vi "WriteData.vi"(8 "error in":errorcluster, 11 "refnum in":refnum<file>) -> (0 "error out":errorcluster, 3 "refnum out":refnum<file>)   [LabVIEW 2017]
doc: "Logs data to csv file on roborio"
uses:
  Robot Global Data.vi
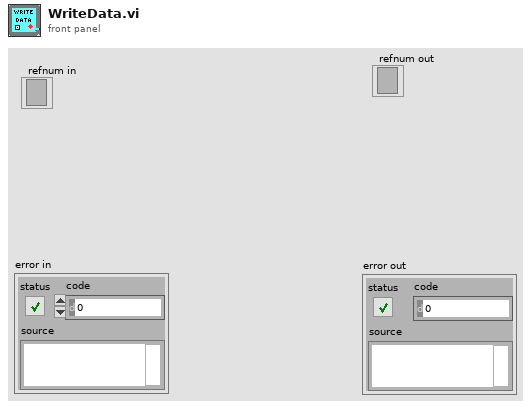
[diagram p1: front panel]
types:
  T1 = typedef "WPI_DriverStationRobotMode2.ctl" = enum16{"Autonomous Disabled", "Autonomous Enabled", "Teleop Disabled", "Teleop Enabled", "Disconnected", "Finish", "Test Disabled", "Test Enabled", "Emergency Stopped"}
  T2 = typedef "Z900_navX_Flags_OpStatusTypeDef.ctl" = u8
  T3 = typedef "Z900_navX_Flags_CalibrationStatusTypeDef.ctl" = u8
  T4 = cluster{"Update Rate Hz":u8, "Accelerometer Full-Scale Range":u8, "Gyro Full-Scale Range":u16, "OP Status":T2, "Calibration Status":T3, "Sensor Status":cluster{"MOVING":bool, "YAW_STABLE":bool, "MAG_DISTURBANCE":bool, "ALTITUDE_VALID":bool, "SEALEVEL_PRESS_SET":bool, "FUSED_HEADING_VALID":bool}, "Self Test Status":cluster{"Gyro Passed":bool, "Accel Passed":bool, "Mag Passed":bool, "Baro Passed":bool, "Complete":bool}}
  T5 = cluster{"Yaw":dbl, "Roll":dbl, "Pitch":dbl, "Heading":dbl, "Fused Heading":dbl}
  T6 = cluster{"LinearAcceleration X":dbl, "LinearAcceleration Y":dbl, "LinearAcceleration Z":dbl}
  T7 = cluster{"MOVING":bool, "YAW_STABLE":bool, "MAG_DISTURBANCE":bool, "ALTITUDE_VALID":bool, "SEALEVEL_PRESS_SET":bool, "FUSED_HEADING_VALID":bool}
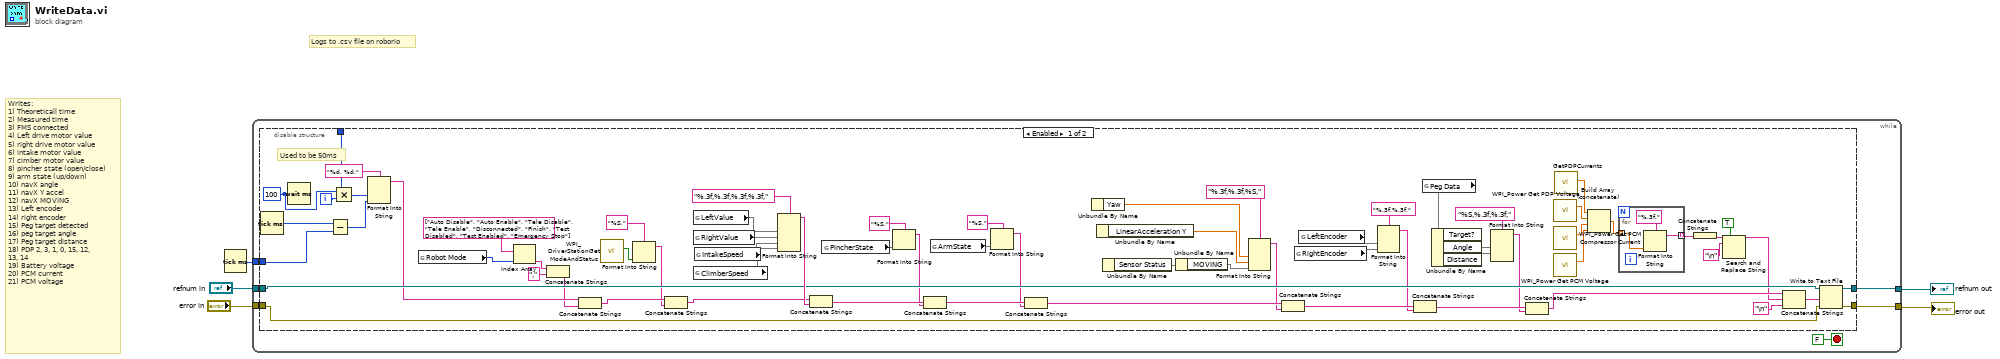
[diagram p0: block diagram]
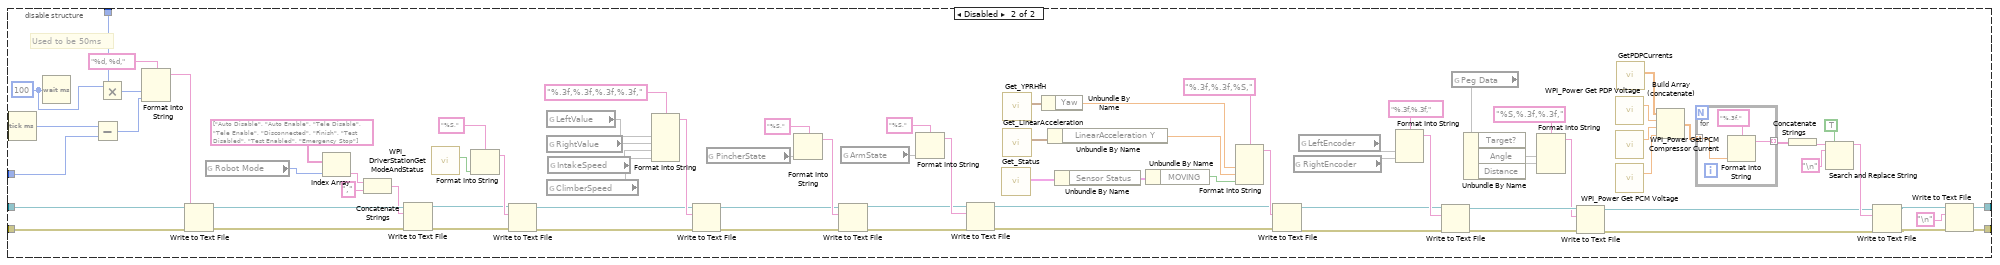
[diagram p2: hidden frame]
diagram:
  # "Logs to .csv file on roborio"
  # "Writes:\n1) Theoreticall time\n2) Measured time\n3) FMS connected\n4) Left drive motor value\n5) right drive motor value\n6) intake motor value\n7) cimber motor value\n8) pincher state (open/close)\n9) arm state (up/down)\n10) navX angle\n11) navX Y accel\n12) navX MOVING\n13) Left encoder\n14) right encoder\n15) Peg target detected\n16) peg target angle\n17) Peg target distance\n18) PDP 2, 3, 1, 0, 15, 12,\n13, 14\n19) Battery voltage\n20) PCM current\n21) PCM voltage"
  n1 = Tick Count (ms)() -> (millisecond timer value=w1:u32)
  n2 = while {
    tunnel: "error in" -> [w10]
    tunnel: "refnum in" -> [w9]
    tunnel: [w7] -> w3
    tunnel: [w8] -> w2
    tunnel: w1 -> [w6]
    i -> [w11]
    stop <- FALSE stop-if-true
    n3 = disable-structure shown="Enabled" {
      disable-tunnel: w11 -> [w80 w165]
      disable-tunnel: w10 -> [w30 w162]
      disable-tunnel: w9 -> [w31 w161]
      disable-tunnel: [w65 w139] -> w8
      disable-tunnel: [w64 w138] -> w7
      disable-tunnel: w6 -> [w37 w87]
      frame Enabled {
        w81 = u32 100 ("milliseconds to wait")
        # "Used to be 50ms"
        n4 = Tick Count (ms)() -> (millisecond timer value=w36:u32)
        n5 = Wait (ms)(milliseconds to wait=w81) -> ()  [unwired: 1 out]
        n6 = Subtract(x=w36, y=w37) -> (x-y=w35:u32)
        n7 = Multiply(x=w81, y=w80) -> (x*y=w79:u32)
        n8 = Format Into String(format string="%d, %d,", w79, w35) -> (resulting string=w29:string)  [unwired: 2 in, 1 out]
        n9 = global read "Robot Global Data.vi" "Robot Mode"() -> (w77:T1)
        n10 = Index Array(array=string[] ["Auto Disable", "Auto Enable", "Tele Disable", "Tele Enable", "Disconnected", "Finish", "Test Disabled", "Test Enabled", "Emergency Stop"], index=w77) -> (element=w56:string)
        n11 = Concatenate Strings(w56, "," ("string")) -> (w28:string)
        n12 = Concatenate Strings(w29, w28) -> (w27:string)
        n13 = call <vilib>:"WPI_DriverStationGetModeAndStatus.vi"() -> ("FMS Attached"=w52:bool)  [unwired: 10 in, 1 out]
        n14 = Format Into String(format string="%S,", w52) -> (resulting string=w26:string)  [unwired: 2 in, 1 out]
        n15 = Concatenate Strings(w27, w26) -> (w25:string)
        n16 = global read "Robot Global Data.vi" "LeftValue"() -> (w75)
        n17 = global read "Robot Global Data.vi" "RightValue"() -> (w74)
        n18 = global read "Robot Global Data.vi" "ClimberSpeed"() -> (w47)
        n19 = global read "Robot Global Data.vi" "IntakeSpeed"() -> (w48)
        n20 = Format Into String(format string="%.3f,%.3f,%.3f,%.3f,", w75, w74, w48, w47) -> (resulting string=w34:string)  [unwired: 2 in, 1 out]
        n21 = Concatenate Strings(w25, w34) -> (w24:string)
        n22 = global read "Robot Global Data.vi" "PincherState"() -> (w44)
        n23 = Format Into String(format string="%S,", w44) -> (resulting string=w23:string)  [unwired: 2 in, 1 out]
        n24 = Concatenate Strings(w24, w23) -> (w22:string)
        n25 = global read "Robot Global Data.vi" "ArmState"() -> (w45)
        n26 = Format Into String(format string="%S,", w45) -> (resulting string=w21:string)  [unwired: 2 in, 1 out]
        n27 = Concatenate Strings(w22, w21) -> (w20:string)
        n28 = Unbundle By Name() -> ("Yaw"=w49:dbl)  [unwired: 1 in]
        n29 = Unbundle By Name() -> ("LinearAcceleration Y"=w70:dbl)  [unwired: 1 in]
        n30 = Unbundle By Name() -> (w72:T4, "Sensor Status"=w71)
        n31 = Unbundle By Name(w71) -> ("MOVING"=w69)
        n32 = Format Into String(format string="%.3f,%.3f,%S,", w49, w70, w69) -> (resulting string=w19:string)  [unwired: 2 in, 1 out]
        n33 = Concatenate Strings(w20, w19) -> (w18:string)
        n34 = global read "Robot Global Data.vi" "RightEncoder"() -> (w58)
        n35 = global read "Robot Global Data.vi" "LeftEncoder"() -> (w57)
        n36 = Format Into String(format string="%.3f,%.3f,", w57, w58) -> (resulting string=w17:string)  [unwired: 2 in, 1 out]
        n37 = Concatenate Strings(w18, w17) -> (w16:string)
        n38 = global read "Robot Global Data.vi" "Peg Data"() -> (w42)
        n39 = Unbundle By Name(w42) -> ("Target?"=w41, "Angle"=w40, "Distance"=w39)
        n40 = Format Into String(format string="%S,%.3f,%.3f,", w41, w40, w39) -> (resulting string=w15:string)  [unwired: 2 in, 1 out]
        n41 = Concatenate Strings(w16, w15) -> (w14:string)
        n42 = call <vilib>:"WPI_Power Get PDP Voltage.vi"() -> ("voltage (V)"=w63:dbl)  [unwired: 14 in, 1 out]
        n43 = call <vilib>:"WPI_Power Get PCM Compressor Current.vi"() -> ("current (A)"=w54:dbl)  [unwired: 14 in, 1 out]
        n44 = call <vilib>:"WPI_Power Get PCM Voltage.vi"() -> ("Input Voltage"=w53:dbl)  [unwired: 13 in, 2 out]
        n45 = call "GetPDPCurrents.vi"() -> ("PDP Currents"=w50:dbl[])  [unwired: 11 in]
        n46 = Build Array (concatenate)(w50, w63, w54, w53) -> (w62:dbl[])
        n47 = for {
          tunnel: w62 -> [w84] mode=indexing
          tunnel: [w82] -> w61 mode=indexing
          n48 = Format Into String(format string="%.3f,", w84) -> (resulting string=w82:string)  [unwired: 2 in, 1 out]
        }
        n49 = Concatenate Strings(w61) -> (w60:string)
        n50 = Search and Replace String(replace all?=TRUE ("replace all? (F)"), input string=w60, search string="\n") -> (result string=w13:string)  [unwired: 5 in, 3 out]
        n51 = Concatenate Strings(w14, w13, "\n") -> (w33:string)
        n52 = Write to Text File(file (use dialog)=w31, text=w33, error in=w30) -> (refnum out=w64:refnum<file>, error out=w65:errorcluster)  [unwired: 1 in, 1 out]
      }
      frame Disabled {
        w166 = u32 100 ("milliseconds to wait")
        # "Used to be 50ms"
        n53 = Tick Count (ms)() -> (millisecond timer value=w86:u32)
        n54 = Wait (ms)(milliseconds to wait=w166) -> ()  [unwired: 1 out]
        n55 = Subtract(x=w86, y=w87) -> (x-y=w85:u32)
        n56 = Multiply(x=w166, y=w165) -> (x*y=w164:u32)
        n57 = Format Into String(format string="%d, %d,", w164, w85) -> (resulting string=w156:string)  [unwired: 2 in, 1 out]
        n58 = Write to Text File(file (use dialog)=w161, text=w156, error in=w162) -> (refnum out=w158:refnum<file>, error out=w157:errorcluster)  [unwired: 1 in, 1 out]
        n59 = global read "Robot Global Data.vi" "Robot Mode"() -> (w160:T1)
        n60 = Index Array(array=string[] ["Auto Disable", "Auto Enable", "Tele Disable", "Tele Enable", "Disconnected", "Finish", "Test Disabled", "Test Enabled", "Emergency Stop"], index=w160) -> (element=w128:string)
        n61 = Concatenate Strings(w128, "," ("string")) -> (w126:string)
        n62 = Write to Text File(file (use dialog)=w158, text=w126, error in=w157) -> (refnum out=w120:refnum<file>, error out=w119:errorcluster)  [unwired: 1 in, 1 out]
        n63 = call <vilib>:"WPI_DriverStationGetModeAndStatus.vi"() -> ("FMS Attached"=w123:bool)  [unwired: 10 in, 1 out]
        n64 = Format Into String(format string="%S,", w123) -> (resulting string=w121:string)  [unwired: 2 in, 1 out]
        n65 = Write to Text File(file (use dialog)=w120, text=w121, error in=w119) -> (refnum out=w118:refnum<file>, error out=w117:errorcluster)  [unwired: 1 in, 1 out]
        n66 = global read "Robot Global Data.vi" "LeftValue"() -> (w155)
        n67 = global read "Robot Global Data.vi" "RightValue"() -> (w154)
        n68 = global read "Robot Global Data.vi" "ClimberSpeed"() -> (w112)
        n69 = global read "Robot Global Data.vi" "IntakeSpeed"() -> (w113)
        n70 = Format Into String(format string="%.3f,%.3f,%.3f,%.3f,", w155, w154, w113, w112) -> (resulting string=w153:string)  [unwired: 2 in, 1 out]
        n71 = Write to Text File(file (use dialog)=w118, text=w153, error in=w117) -> (refnum out=w103:refnum<file>, error out=w102:errorcluster)  [unwired: 1 in, 1 out]
        n72 = global read "Robot Global Data.vi" "PincherState"() -> (w105)
        n73 = Format Into String(format string="%S,", w105) -> (resulting string=w111:string)  [unwired: 2 in, 1 out]
        n74 = Write to Text File(file (use dialog)=w103, text=w111, error in=w102) -> (refnum out=w109:refnum<file>, error out=w108:errorcluster)  [unwired: 1 in, 1 out]
        n75 = global read "Robot Global Data.vi" "ArmState"() -> (w106)
        n76 = Format Into String(format string="%S,", w106) -> (resulting string=w110:string)  [unwired: 2 in, 1 out]
        n77 = Write to Text File(file (use dialog)=w109, text=w110, error in=w108) -> (refnum out=w101:refnum<file>, error out=w100:errorcluster)  [unwired: 1 in, 1 out]
        n78 = call <vilib>:"Get_Status.vi"() -> ("Status"=w150:T4)  [unwired: 11 in]
        n79 = call <vilib>:"Get_YPRHfH.vi"() -> ("YRPHfH"=w115:T5)  [unwired: 11 in]
        n80 = call <vilib>:"Get_LinearAcceleration.vi"() -> ("Linear Acceleration"=w151:T6)  [unwired: 11 in]
        n81 = Unbundle By Name(w115) -> ("Yaw"=w114:dbl)
        n82 = Unbundle By Name(w151) -> ("LinearAcceleration Y"=w148:dbl)
        n83 = Unbundle By Name(w150) -> ("Sensor Status"=w149:T7)
        n84 = Unbundle By Name(w149) -> ("MOVING"=w147:bool)
        n85 = Format Into String(format string="%.3f,%.3f,%S,", w114, w148, w147) -> (resulting string=w145:string)  [unwired: 2 in, 1 out]
        n86 = Write to Text File(file (use dialog)=w101, text=w145, error in=w100) -> (refnum out=w143:refnum<file>, error out=w142:errorcluster)  [unwired: 1 in, 1 out]
        n87 = global read "Robot Global Data.vi" "RightEncoder"() -> (w130)
        n88 = global read "Robot Global Data.vi" "LeftEncoder"() -> (w129)
        n89 = Format Into String(format string="%.3f,%.3f,", w129, w130) -> (resulting string=w144:string)  [unwired: 2 in, 1 out]
        n90 = Write to Text File(file (use dialog)=w143, text=w144, error in=w142) -> (refnum out=w97:refnum<file>, error out=w96:errorcluster)  [unwired: 1 in, 1 out]
        n91 = global read "Robot Global Data.vi" "Peg Data"() -> (w95)
        n92 = Unbundle By Name(w95) -> ("Target?"=w94, "Angle"=w93, "Distance"=w92)
        n93 = Format Into String(format string="%S,%.3f,%.3f,", w94, w93, w92) -> (resulting string=w90:string)  [unwired: 2 in, 1 out]
        n94 = Write to Text File(file (use dialog)=w97, text=w90, error in=w96) -> (refnum out=w89:refnum<file>, error out=w88:errorcluster)  [unwired: 1 in, 1 out]
        n95 = call <vilib>:"WPI_Power Get PDP Voltage.vi"() -> ("voltage (V)"=w136:dbl)  [unwired: 14 in, 1 out]
        n96 = call <vilib>:"WPI_Power Get PCM Compressor Current.vi"() -> ("current (A)"=w125:dbl)  [unwired: 14 in, 1 out]
        n97 = call <vilib>:"WPI_Power Get PCM Voltage.vi"() -> ("Input Voltage"=w124:dbl)  [unwired: 13 in, 2 out]
        n98 = call "GetPDPCurrents.vi"() -> ("PDP Currents"=w116:dbl[])  [unwired: 11 in]
        n99 = Build Array (concatenate)(w116, w136, w125, w124) -> (w135:dbl[])
        n100 = for {
          tunnel: w135 -> [w169] mode=indexing
          tunnel: [w167] -> w134 mode=indexing
          n101 = Format Into String(format string="%.3f,", w169) -> (resulting string=w167:string)  [unwired: 2 in, 1 out]
        }
        n102 = Concatenate Strings(w134) -> (w133:string)
        n103 = Search and Replace String(replace all?=TRUE ("replace all? (F)"), input string=w133, search string="\n") -> (result string=w132:string)  [unwired: 5 in, 3 out]
        n104 = Write to Text File(file (use dialog)=w89, text=w132, error in=w88) -> (refnum out=w99:refnum<file>, error out=w98:errorcluster)  [unwired: 1 in, 1 out]
        n105 = Write to Text File(file (use dialog)=w99, text="\n", error in=w98) -> (refnum out=w138:refnum<file>, error out=w139:errorcluster)  [unwired: 1 in, 1 out]
      }
    }
  }
  "refnum out" <- w3
  "error out" <- w2
